vi "Read Message.vi"(0 "Rx Com Udp Port":T1 {"Handle" format="%08x"}, 5 "Channel Index":i32, 11 "error in (no error)":errorcluster) -> (4 "data buffer out":u8[](array[numeric]), 6 "status data out":u32[](array[numeric]), 8 "Data Available":bool, 15 "error out":errorcluster)   [LabVIEW 2013, in "AIT 664 Custom Device.lvlib"]
doc: "Read data and status from the AIT 664 card."
uses:
  AIT 664 Custom Device.lvlib
  <userlib>/ARINC 664/AIT 664 Controls/General/Message Port.ctl
  <userlib>/ARINC 664/AIT 664 Controls/General/Direction.ctl
  <userlib>/ARINC 664/AIT 664 Controls/General/Message Port Type.ctl
  <instrlib>/AIT 664/Private/AIT 664 Data/Rx/Read/AIT 664 Rx Read (ComUdp).vi
  <instrlib>/AIT 664/AIT 664.lvlib
  <vilib>/NI Veristand/Custom Device Tools/Custom Device Utility Library/Custom Device Utility Library.lvlib
  <userlib>/ARINC 664/AIT 664 API.lvlib
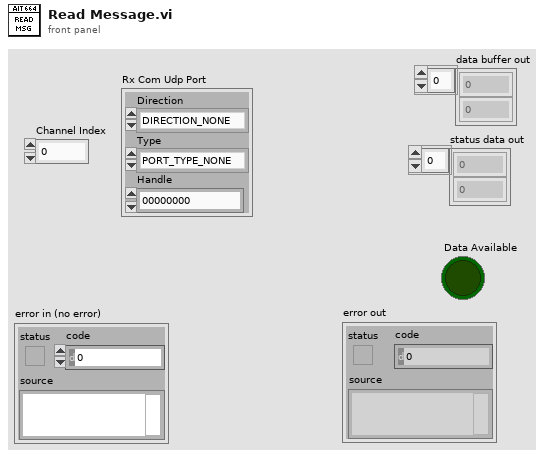
[diagram p1: front panel]
types:
  T1 = typedef "AIT 664 API.lvlib/Message Port.ctl" = cluster{"Direction":T2, "Type":T3, "Handle":u64}
  T2 = typedef "AIT 664 API.lvlib/Direction.ctl" = enum16{"DIRECTION_NONE", "DIRECTION_TX", "DIRECTION_RX"}
  T3 = typedef "AIT 664 API.lvlib/Message Port Type.ctl" = enum16{"PORT_TYPE_NONE", "COM_UDP", "SAP_UDP", "SAP_IP", "SAP_MAC", "COTS_MAC", "COTS_MAC_RAW"}
  T4 = cluster{"Day":u32, "Hour":u32, "Min.":u32, "Sec.":u32, "Nanosecond":u32}
  T5 = typedef "AIT 664 API.lvlib/Com Udp Read Data.ctl" = cluster{"Rx Com Udp Data":u8[], "Network Interface":T6}
  T6 = typedef "AIT 664 API.lvlib/Network Interface.ctl" = enum32{"Network_A", "Network_B"}
  T7 = typedef "AIT 664 API.lvlib/Rx Message Port Status.ctl" = cluster{"Rx Message Port Type":T8, "Port ID":u32, "ES Index":u32, "Valid Message Count":u32, "Invalid Message Count":u32, "No Buffer Available Error Count":u32, "Num Empty Buffers":u16, "Num Full Buffers":u16}
  T8 = typedef "AIT 664 API.lvlib/Rx Message Port Type.ctl" = u32
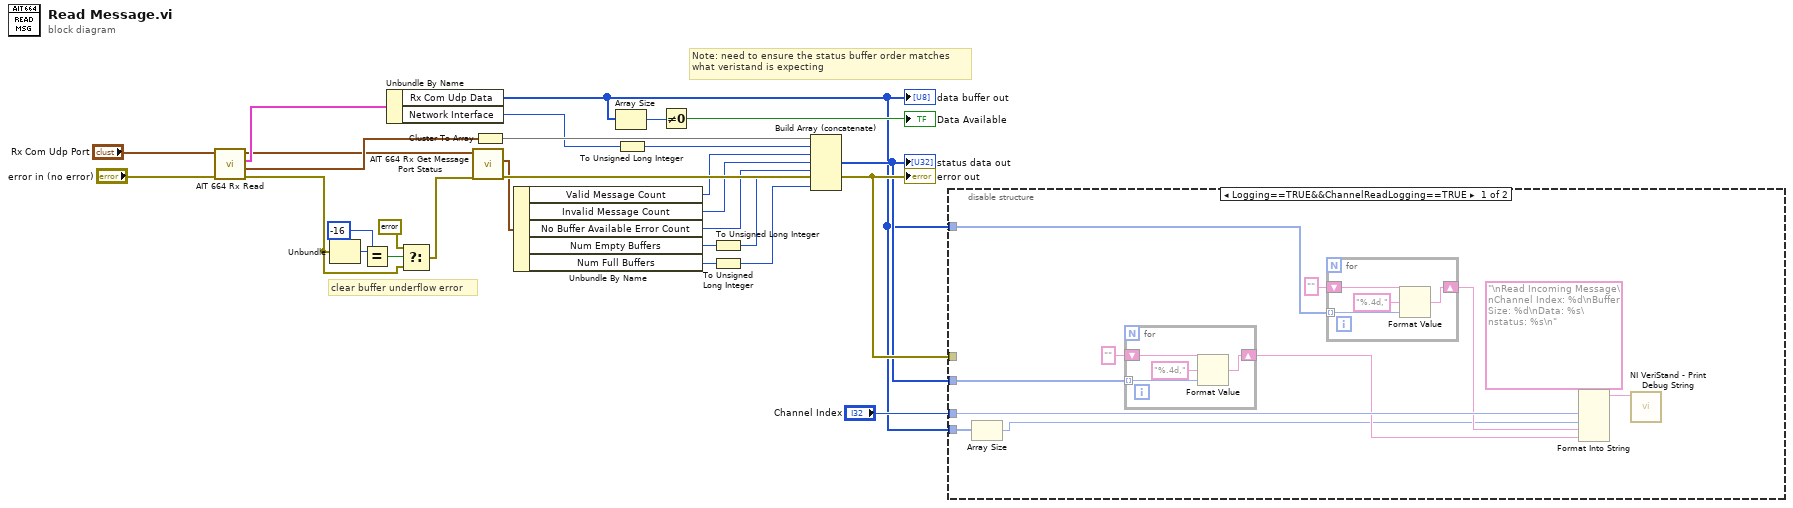
[diagram p0: block diagram]
diagram:
  # "Note: need to ensure the status buffer order matches\nwhat veristand is expecting"
  # "clear buffer underflow error"
  n1 = call-poly <instrlib>:"AIT 664 Rx Read.vi"("error in"="error in (no error)", "Rx Com Udp Port in"="Rx Com Udp Port") -> ("error out"=w3:errorcluster, "Time Stamp"=w21:T4, "Com Udp Read Data out"=w22:T5, "Rx Com Udp Port out"=w19:T1)  [unwired: 4 in]
  n2 = Unbundle(w3) -> ("code"=w8:i32)  [unwired: 2 out]
  n3 = Equal?(x=w8, y=-16) -> (x = y?=w6:bool)
  n4 = Unbundle By Name(w22) -> ("Rx Com Udp Data"=w1:u8[], "Network Interface"=w16:T6)
  "data buffer out" <- w1
  n5 = Select(t=errorcluster {"status"=FALSE, "code"=0, "source"=""} ("error out"), s=w6, f=w3) -> (s? t:f=w5:errorcluster)
  n6 = call <instrlib>:"AIT 664 Rx Get Message Port Status.vi"("error in"=w5, "Rx Port in"=w19) -> ("error out"=w20:errorcluster, "Rx Message Port Status out"=w18:T7)  [unwired: 5 in, 1 out]
  "error out" <- w20
  n7 = Cluster To Array(cluster=w21) -> (array=w17:u32[])
  n8 = Unbundle By Name(w18) -> ("Valid Message Count"=w15:u32, "Invalid Message Count"=w14:u32, "No Buffer Available Error Count"=w13:u32, "Num Empty Buffers"=w12:u16, "Num Full Buffers"=w10:u16)
  n9 = Array Size(array=w1) -> (size(s)=w27:i32)
  n10 = To Unsigned Long Integer(number=w16) -> (unsigned 32bit integer=w26:u32)
  n11 = Not Equal To 0?(x=w27) -> (x != 0?=→"Data Available":bool)
  n12 = To Unsigned Long Integer(number=w12) -> (unsigned 32bit integer=w11:u32)
  n13 = To Unsigned Long Integer(number=w10) -> (unsigned 32bit integer=w9:u32)
  n14 = Build Array (concatenate)(w17, w26, w15, w14, w13, w11, w9) -> (w2:u32[])
  "status data out" <- w2
  n15 = disable-structure shown="Logging==TRUE&&ChannelReadLogging==TRUE" {
    disable-tunnel: w1 -> [w39 _]
    disable-tunnel: "Channel Index" -> [w36 _]
    disable-tunnel: w20 -> [_ _]
    disable-tunnel: w2 -> [w32 _]
    disable-tunnel: w1 -> [w30 _]
    frame condition #0 {
      n16 = Array Size(array=w30) -> (size(s)=w29:i32)
      n17 = for {
        tunnel: w32 -> [w40] mode=indexing
        shift-right: [w41] -> w31
        shift-left: "" ("output string") -> [w42]
        n18 = Format Value(string ("")=w42, format string="%.4d,", value (0)=w40) -> (output string=w41:string)
      }
      n19 = for {
        tunnel: w39 -> [w44] mode=indexing
        shift-right: [w45] -> w35
        shift-left: "" ("format string") -> [w46]
        n20 = Format Value(string ("")=w46, format string="%.4d,", value (0)=w44) -> (output string=w45:string)
      }
      n21 = Format Into String(format string="\nRead Incoming Message\nChannel Index: %d\nBuffer Size: %d\nData: %s\nstatus: %s\n", w36, w29, w35, w31) -> (resulting string=w34:string)  [unwired: 2 in, 1 out]
      n22 = call <vilib>:"NI VeriStand - Print Debug String.vi"("Message"=w34) -> ()  [unwired: 10 in, 1 out]
    }
    frame condition #1 (active) {
    }
  }
